vi "Array_Trans.vi"(0 "RB01":dbl[](array[numeric]), 1 "Array 8":dbl[](array[numeric]), 5 "Kappa 2":dbl[](array[numeric]), 7 "RB01 2":dbl[](array[numeric]), 9 "Tau 2":dbl[](array[numeric]), 12 "Kappa":dbl[](array[numeric]), 13 "Tau":dbl[](array[numeric])) -> (2 "Array 7":dbl[][](array[numeric]), 3 "Array 4":dbl[][](array[numeric]), 4 "Array":dbl[][](array[numeric]), 6 "Array 3":dbl[][](array[numeric]), 8 "Array 6":dbl[][](array[numeric]), 10 "Array 2":dbl[][](array[numeric]), 14 "Array 5":dbl[][](array[numeric]))   [LabVIEW 2014]
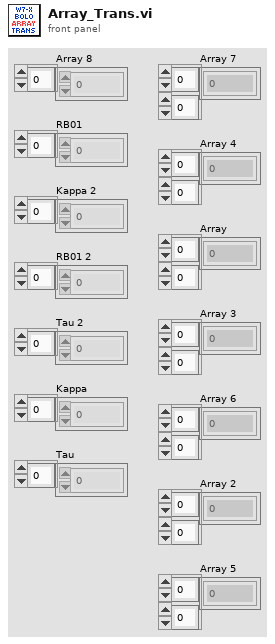
[diagram p1: front panel]
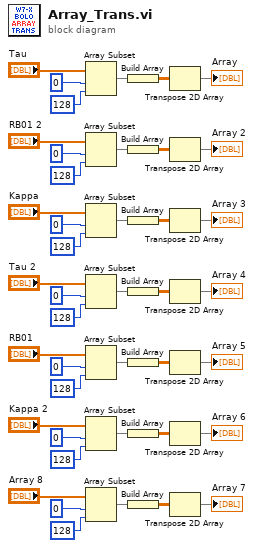
[diagram p0: block diagram]
diagram:
  n1 = Array Subset(array="Tau", index=0, length=128) -> (w39:dbl[])
  n2 = Array Subset(array="RB01 2", index=0, length=128) -> (w36:dbl[])
  n3 = Array Subset(array="Kappa", index=0, length=128) -> (w32:dbl[])
  n4 = Array Subset(array="Tau 2", index=0, length=128) -> (w29:dbl[])
  n5 = Array Subset(array="RB01", index=0, length=128) -> (w27:dbl[])
  n6 = Array Subset(array="Kappa 2", index=0, length=128) -> (w24:dbl[])
  n7 = Array Subset(array="Array 8", index=0, length=128) -> (w17:dbl[])
  n8 = Build Array(w39) -> (w38:dbl[][])
  n9 = Build Array(w36) -> (w35:dbl[][])
  n10 = Build Array(w32) -> (w33:dbl[][])
  n11 = Build Array(w29) -> (w30:dbl[][])
  n12 = Build Array(w27) -> (w26:dbl[][])
  n13 = Build Array(w24) -> (w25:dbl[][])
  n14 = Build Array(w17) -> (w21:dbl[][])
  n15 = Transpose 2D Array(2D array=w38) -> (transposed array=→"Array":dbl[][])
  n16 = Transpose 2D Array(2D array=w35) -> (transposed array=→"Array 2":dbl[][])
  n17 = Transpose 2D Array(2D array=w33) -> (transposed array=→"Array 3":dbl[][])
  n18 = Transpose 2D Array(2D array=w30) -> (transposed array=→"Array 4":dbl[][])
  n19 = Transpose 2D Array(2D array=w26) -> (transposed array=→"Array 5":dbl[][])
  n20 = Transpose 2D Array(2D array=w25) -> (transposed array=→"Array 6":dbl[][])
  n21 = Transpose 2D Array(2D array=w21) -> (transposed array=→"Array 7":dbl[][])
